vi "sub_calDistanceVLP16.vi"(9 "Index (Channel)":i32, 10 "Index (Firing Sequence)":i32, 11 "Byte Array":u8[](array[numeric])) -> (3 "distance (meter)":dbl)   [LabVIEW 2020]
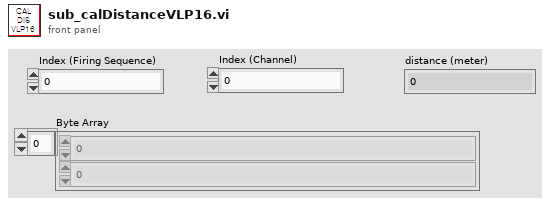
[diagram p1: front panel]
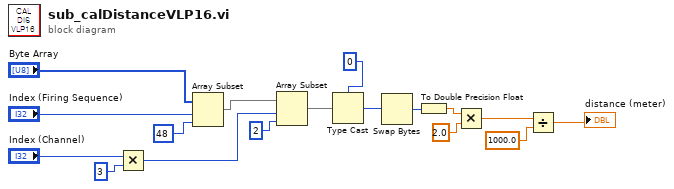
[diagram p0: block diagram]
diagram:
  n1 = Multiply(x="Index (Channel)", y=3) -> (x*y=w10:i32)
  n2 = Array Subset(array="Byte Array", index="Index (Firing Sequence)", length=48 ("길이")) -> (w7:u8[])
  n3 = Array Subset(array=w7, index=w10, length=2 ("길이")) -> (w17:u8[])
  n4 = Type Cast(type=u16 0, x=w17) -> (*(type *) &x=w13:u16)
  n5 = Swap Bytes(anything=w13) -> (byte swapped=w14:u16)
  n6 = To Double Precision Float(number=w14) -> (double precision float=w15:dbl)
  n7 = Multiply(x=w15, y=2.0) -> (x*y=w3:dbl)
  n8 = Divide(x=w3, y=1000.0) -> (x/y=→"distance (meter)":dbl)
